vi "getMessage.vi"(8 "error in (no error)":errorcluster, 11 "TCPClient in":refnum<class "TCPClient.lvclass">) -> (0 "error out":errorcluster, 2 "String":string, 3 "TCPClient out":refnum<class "TCPClient.lvclass">)   [LabVIEW 2016, in "TCPClient.lvclass"]
uses:
  TCPClient.lvclass
  home/plotz/lsst_ts/ss_atDome/common_labview_tcpdevice/ts_labview_tcp/TCPCommunicator/TCPCommunicator.lvclass
  TCPCommunicator/TCPCommunicator.lvclass/TCPCommunicator.ctl
  TCPSettings/TCPSettings.lvclass
  TCPCommunicator/TCPCommunicator.lvclass
  TCPComEvents/TCPComEvents.lvclass
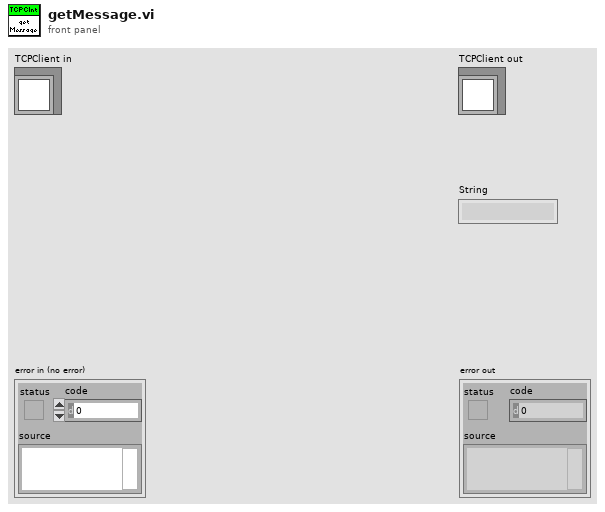
[diagram p1: front panel]
types:
  T1 = enum16{"Standard", "Buffered", "CRLF", "Immediate"}
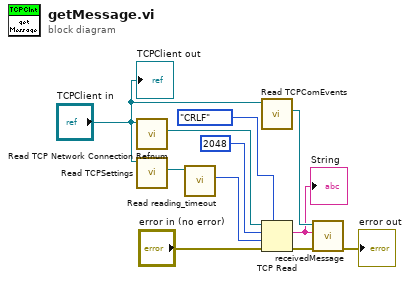
[diagram p0: block diagram]
diagram:
  n1 = call-dynamic "Read TCP Network Connection Refnum.vi"("TCPCommunicator in"="TCPClient in") -> ("TCP Network Connection Refnum"=w8:refnum<k5>)  [unwired: 8 in, 2 out]
  n2 = call-dynamic "Read TCPSettings.vi"("TCPCommunicator in"="TCPClient in") -> ("TCPSettings.lvclass"=w7:refnum<class "TCPSettings.lvclass">)  [unwired: 8 in, 2 out]
  n3 = call-dynamic "Read reading_timeout.vi"("TCPSettings in"=w7) -> ("reading_timeout"=w9:i32)  [unwired: 8 in, 2 out]
  n4 = call "Read TCPComEvents.vi"("TCPCommunicator in"="TCPClient in") -> ("TCPComEvents.lvclass"=w11:refnum<class "TCPComEvents.lvclass">)  [unwired: 8 in, 2 out]
  n5 = TCP Read(connection ID=w8, bytes to read=2048, error in (no error)="error in (no error)", 7:T1."CRLF" ("mode (standard)"), 9:w9) -> (data out=w4:string, error out=w10:errorcluster)  [unwired: 1 out]
  "String" <- w4
  n6 = call "receivedMessage.vi"("error in (no error)"=w10, "message"=w4, "TCPComEvents in"=w11) -> ("error out"=→"error out":errorcluster)  [unwired: 7 in, 1 out]
  "TCPClient out" <- "TCPClient in"
